vi "ma_single_Check Time Signal Continuity (CDB).vi"(5 "Ignore input time stamp":bool, 8 "error in (no error)":errorcluster, 11 "Waveform":waveform(cdb)={"t0"=timestamp(0 s since 1904-01-01), "dt"=0.0, "Y"=[]}) -> (0 "error out":errorcluster, 1 "epsilon used":dbl format="%0.2f", 2 "dt changed":bool, 3 "t0 changed":bool)   [LabVIEW 2020, in "NI_MABase.lvlib"]
uses:
  NI_MABase.lvlib
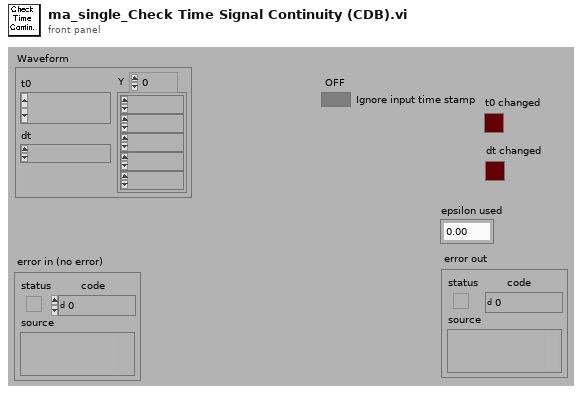
[diagram p1: front panel]
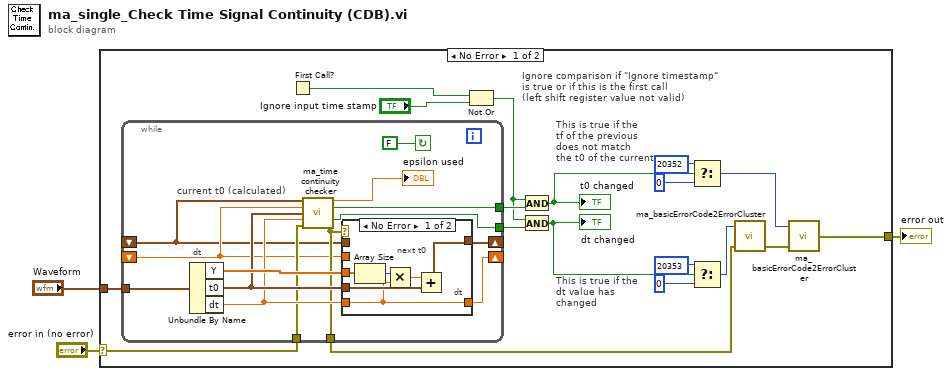
[diagram p0: block diagram]
diagram:
  n1 = case shown="No Error" "error in (no error)" {
    selector: "error in (no error)" -> [w6 w44]
    tunnel: [w10 w44] -> w2
    tunnel: "Waveform" -> [w4 _]
    frame No Error {
      # "Ignore comparison if \"Ignore timestamp\" \nis true or if this is the first call \n(left shift register value not valid)"
      # "This is true if the\ntf of the previous\ndoes not match \nthe t0 of the current"
      # "This is true if the\ndt value has \nchanged"
      n2 = while {
        tunnel: [w28] -> w21
        tunnel: [w29] -> w20
        shift-left: _ -> [w24]
        shift-right: [w26] -> _
        shift-left: _ -> [w23]
        shift-right: [w35] -> _
        tunnel: w6 -> [w27]
        tunnel: [w25] -> w5
        tunnel: w4 -> [w22]
        stop <- FALSE continue-if-true
        # "current t0 (calculated)"
        # "dt"
        n3 = Unbundle By Name(w22) -> ("Y"=w33:cdb[], "t0"=w32:timestamp, "dt"=w31:dbl)
        n4 = call "ma_time continuity checker.vi"("timestamp previous"=w23, "dt previous"=w24, "timestamp current"=w32, "dt current"=w31, "error in (no error)"=w27) -> ("epsilon used"=→"epsilon used":dbl, "t0 changed"=w29:bool, "dt changed"=w28:bool, "error out"=w25:errorcluster)  [unwired: 7 in]
        n5 = case shown="No Error" w25 {
          tunnel: [w41 w42] -> w35
          tunnel: w33 -> [w38 _]
          tunnel: w32 -> [w37 _]
          tunnel: w31 -> [w36 _]
          tunnel: [w36 w43] -> w26
          tunnel: w24 -> [_ w43]
          tunnel: w23 -> [_ w42]
          frame No Error {
            # "dt"
            # "next t0"
            n6 = Array Size(array=w38) -> (size(s)=w40:i32)
            n7 = Multiply(x=w40, y=w36) -> (x*y=w39:dbl)
            n8 = Add(x=w39, y=w37) -> (x+y=w41:timestamp)
          }
          frame Error {
          }
        }
      }
      n9 = First Call?() -> (First Call?: T/F=w7:bool)
      n10 = Not Or(1:"Ignore input time stamp", 2:w7) -> (0:w9:bool)
      n11 = And(x=w9, y=w20) -> (x .and. y?=w19:bool)
      "t0 changed" <- w19
      n12 = And(x=w9, y=w21) -> (x .and. y?=w13:bool)
      "dt changed" <- w13
      n13 = Select(t=20352 ("code"), s=w19, f=0) -> (s? t:f=w16:i32)
      n14 = Select(t=20353 ("code"), s=w13, f=0) -> (s? t:f=w12:i32)
      n15 = call "ma_basicErrorCode2ErrorCluster.vi"("error in (no error)"=w5, "Error Code"=w12) -> ("error out"=w11:errorcluster)  [unwired: 1 in]
      n16 = call "ma_basicErrorCode2ErrorCluster.vi"("error in (no error)"=w11, "Error Code"=w16) -> ("error out"=w10:errorcluster)  [unwired: 1 in]
    }
    frame Error {
    }
  }
  "error out" <- w2
